vi "FGV - event data.vi"(7 "Action (Read)":enum16{"Init", "Read", "Génère", "Supprimer"}(ring)=enum."Read", 8 "entrée d'erreur (pas d'erreur)":errorcluster, 10 "Event Data":cluster{"Position":i32}) -> (0 "sortie d'erreur":errorcluster, 3 "Refnum d'abonnement à des événements":refnum<event-registration>)   [LabVIEW 2019]
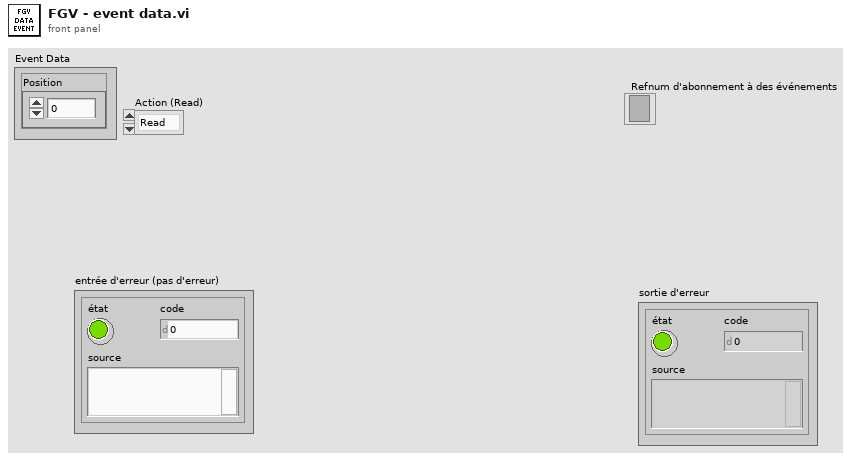
[diagram p1: front panel]
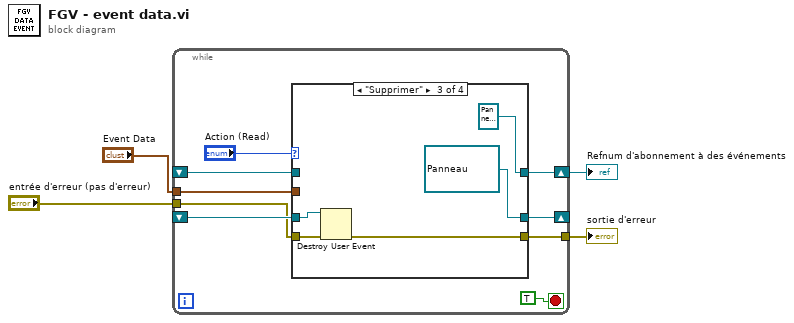
[diagram p0: block diagram]
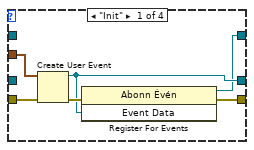
[diagram p2: hidden frame]
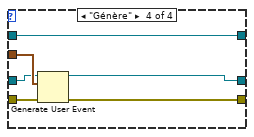
[diagram p4: hidden frame]
diagram:
  n1 = while {
    shift-right: [w11] -> w4
    shift-left: _ -> [w10]
    shift-right: [w12] -> _
    shift-left: _ -> [w9]
    tunnel: "entrée d'erreur (pas d'erreur)" -> [w7]
    tunnel: [w6] -> w2
    tunnel: "Event Data" -> [w5]
    stop <- TRUE stop-if-true
    n2 = case shown="\"Supprimer\"" "Action (Read)" {
      tunnel: [w18 w21 refnum<user-event> refnum ("Event Data") w29] -> w12
      tunnel: [w17 w22 refnum<event-registration> refnum ("Refnum d'abonnement à des événements") w28] -> w11
      tunnel: w10 -> [_ w22 _ w28]
      tunnel: w9 -> [_ w21 w26 w32]
      tunnel: w7 -> [w16 w20 w27 w31]
      tunnel: [w15 w20 w25 w30] -> w6
      tunnel: w5 -> [w14 _ _ w33]
      frame "Init" {
        n3 = Create User Event(user event datatype=w14, error in=w16) -> (user event=w18:refnum<user-event>, error out=w19:errorcluster)
        n4 = register-events(error in=w19, w18) -> (reference out=w17:refnum<event-registration>, error out=w15:errorcluster)  [unwired: 1 in]
      }
      frame "Read", Default {
      }
      frame "Supprimer" {
        n5 = Destroy User Event(user event=w26, error in=w27) -> (error out=w25:errorcluster)
      }
      frame "Génère" {
        n6 = Generate User Event(user event=w32, event data cluster=w33, error in=w31) -> (user event out=w29:refnum<user-event>, error out=w30:errorcluster)  [unwired: 1 in]
      }
    }
  }
  "Refnum d'abonnement à des événements" <- w4
  "sortie d'erreur" <- w2
